vi "GOOP_GetApplicationBasedOnLvClass.vi"(8 "error in (no error)":errorcluster, 11 "LVClassLibrary in":refnum<vi>) -> (0 "error out":errorcluster, 3 "Application out":refnum<vi>)   [LabVIEW 2020]
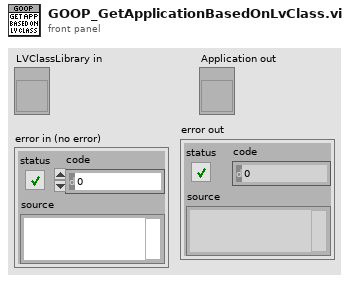
[diagram p1: front panel]
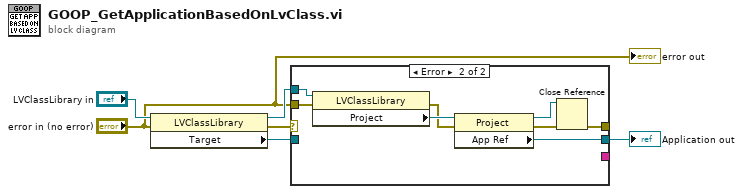
[diagram p0: block diagram]
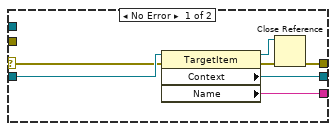
[diagram p2: hidden frame]
diagram:
  n1 = property class="LVClassLibrary"(reference="LVClassLibrary in", error in="error in (no error)") -> (reference out=w6:refnum<vi>, error out=w3:errorcluster, "Target"=w4:refnum<vi>)
  n2 = case shown="Error" w3 {
    selector: w3 -> [w9 _]
    tunnel: w4 -> [w13 _]
    tunnel: [w12 w15] -> w5
    tunnel: [w8 w16] -> _
    tunnel: w6 -> [_ w21]
    tunnel: "error in (no error)" -> [_ w20]
    tunnel: [w7 _] -> _
    frame No Error {
      n3 = property class="TargetItem"(reference=w13, error in=w9) -> (reference out=w10:refnum<vi>, error out=w11:errorcluster, "Context"=w12:refnum<vi>, "Name"=w7:string)
      n4 = Close Reference(reference=w10, error in (no error)=w11) -> (error out=w8:errorcluster)
    }
    frame Error {
      n5 = property class="LVClassLibrary"(reference=w21, error in=w20) -> (error out=w14:errorcluster, "Project"=w19:refnum<vi>)  [unwired: 1 out]
      n6 = property class="Project"(reference=w19, error in=w14) -> (reference out=w17:refnum<vi>, error out=w18:errorcluster, "App Ref"=w15:refnum<vi>)
      n7 = Close Reference(reference=w17, error in (no error)=w18) -> (error out=w16:errorcluster)
    }
  }
  "Application out" <- w5
  "error out" <- "error in (no error)"
